vi "Initialize.vi"(8 "error in":errorcluster, 10 "InstanceName":string, 11 "Chiller Cluster - 2 Channel.lvclass":refnum<class "Climate Chamber - 2 Channel.lvclass">) -> (0 "error out":errorcluster, 3 "output cluster":refnum<class "Climate Chamber - 2 Channel.lvclass">)   [LabVIEW 2023, in "Climate Chamber - 2 Channel.lvclass"]
uses:
  Climate Chamber - 2 Channel.lvclass
  Climate Chamber - 2 Channel.lvclass/Climate Chamber - 2 Channel.ctl
  aa699e23-44e5-4879-a6c3-559a5ef9d2df.vi
  f052ae29-6a80-40ba-948a-362e912d77bd.vi
  293d8571-9b14-4487-9d38-5c4ef123197a.vi
  16278833-8dfa-4f0a-81f5-f65bd27da24d.vi
  da48c8f8-b897-4dcf-9451-5b341042a248.vi
  f0f9fcd1-ad99-4552-afb1-31be6853704b.vi
  aa699e23-44e5-4879-a6c3-559a5ef9d2df.vi/4bc1c15b-36ab-481f-b8dd-c64075ce723a.vi
  f052ae29-6a80-40ba-948a-362e912d77bd.vi/4bc1c15b-36ab-481f-b8dd-c64075ce723a.vi
  293d8571-9b14-4487-9d38-5c4ef123197a.vi/4bc1c15b-36ab-481f-b8dd-c64075ce723a.vi
  16278833-8dfa-4f0a-81f5-f65bd27da24d.vi/4bc1c15b-36ab-481f-b8dd-c64075ce723a.vi
  da48c8f8-b897-4dcf-9451-5b341042a248.vi/4bc1c15b-36ab-481f-b8dd-c64075ce723a.vi
  f0f9fcd1-ad99-4552-afb1-31be6853704b.vi/4bc1c15b-36ab-481f-b8dd-c64075ce723a.vi
  <vilib>/ADAS Replay HIL/Channels/Tag Wrapper/Polymorphic/Open Producer Tag (Cluster).vi
  <vilib>/ADAS Replay HIL/AdasHilServices/AdasHilServices Fill In Error Info Ex.vi
  <vilib>/ADAS Replay HIL/Channels/Tag Wrapper/Polymorphic/Open Consumer Tag (Cluster).vi
  Utilities/Utilities.lvlib
  <vilib>/ADAS Replay HIL/Channels/Tag Wrapper/Tag Wrapper.lvlib
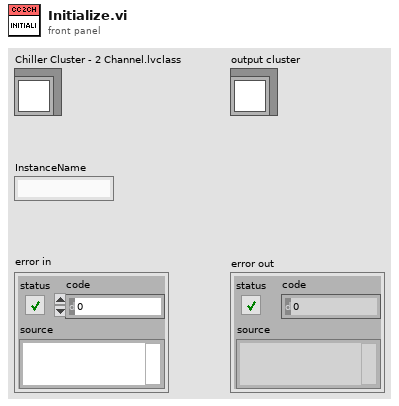
[diagram p1: front panel]
types:
  T1 = cluster{"OnOff.ACT":bool, "ErrorAcknowledge.ACT":bool}
  T2 = cluster{"OnOff.STS":i32, "Error.STS":i32, "Watchdog.STS":i32}
  T3 = cluster{"Temperature.ch01.SP":dbl, "TemperatureMIN.ch01.SP":dbl, "TemperatureMAX.ch01.SP":dbl, "TemperatureGrad.ch01.SP":dbl, "Humidity.ch01.SP":dbl, "HumidityMIN.ch01.SP":dbl, "HumidityMAX.ch01.SP":dbl, "HumidityGrad.ch01.SP":dbl}
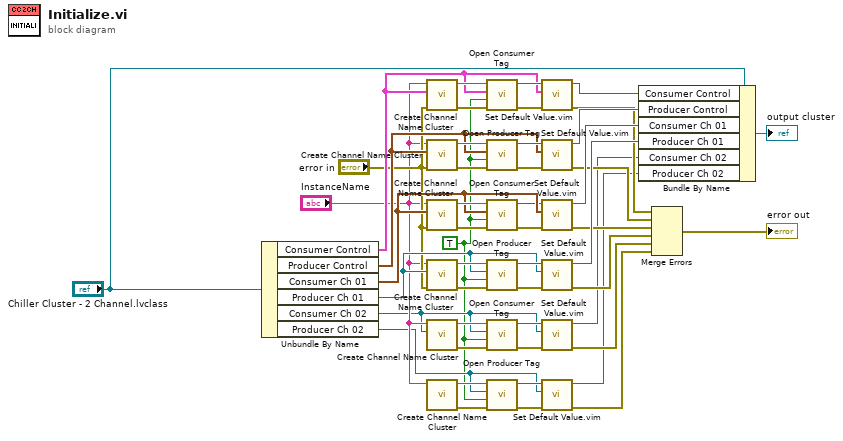
[diagram p0: block diagram]
diagram:
  w6 = TRUE ("Create if not found? (T)")
  n1 = Unbundle By Name("Chiller Cluster - 2 Channel.lvclass") -> ("Consumer Control"=w44:T1, "Producer Control"=w39:T2, "Consumer Ch 01"=w35:T3, "Producer Ch 01"=w31:refnum<k21>, "Consumer Ch 02"=w7:refnum<k21>, "Producer Ch 02"=w10:refnum<k21>)
  n2 = call "Create Channel Name Cluster.vi"("error in"="error in", "Cluster"=w44, "Instance Name"="InstanceName") -> ("error out"=w25:errorcluster, "Data Channel Name"=w48:string)  [unwired: 7 in]
  n3 = call "Create Channel Name Cluster.vi"("error in"="error in", "Cluster"=w39, "Instance Name"="InstanceName") -> ("error out"=w26:errorcluster, "Data Channel Name"=w47:string)  [unwired: 7 in]
  n4 = call "Create Channel Name Cluster.vi"("error in"="error in", "Cluster"=w35, "Instance Name"="InstanceName") -> ("error out"=w32:errorcluster, "Data Channel Name"=w38:string)  [unwired: 7 in]
  n5 = call "Create Channel Name Cluster.vi"("error in"="error in", "Cluster"=w31, "Instance Name"="InstanceName") -> ("error out"=w29:errorcluster, "Data Channel Name"=w37:string)  [unwired: 7 in]
  n6 = call "Create Channel Name Cluster.vi"("Cluster"=w7, "Instance Name"="InstanceName") -> ("error out"=w14:errorcluster, "Data Channel Name"=w9:string)  [unwired: 8 in]
  n7 = call "Create Channel Name Cluster.vi"("Instance Name"="InstanceName") -> ("error out"=w12:errorcluster, "Data Channel Name"=w17:string)  [unwired: 9 in]
  n8 = call-poly <vilib>:"Open Consumer Tag.vi"("error in"=w25, "Create if not found? (T)"=w6, "Cluster"=w44, "Channel Name"=w48) -> ("error out"=w43:errorcluster, "ADAS HIL Channel"=w46:refnum<k21>)  [unwired: 6 in]
  n9 = call-poly <vilib>:"Open Producer Tag.vi"("error in"=w26, "Create if not found? (T)"=w6, "Cluster"=w39, "Channel Name"=w47) -> ("error out"=w42:errorcluster, "ADAS HIL Channel"=w41:refnum<k21>)  [unwired: 6 in]
  n10 = call-poly <vilib>:"Open Consumer Tag.vi"("error in"=w32, "Create if not found? (T)"=w6, "Cluster"=w35, "Channel Name"=w38) -> ("error out"=w33:errorcluster, "ADAS HIL Channel"=w34:refnum<k21>)  [unwired: 6 in]
  n11 = call-poly <vilib>:"Open Producer Tag.vi"("error in"=w29, "Create if not found? (T)"=w6, "Cluster"=w31, "Channel Name"=w37) -> ("error out"=w30:errorcluster, "ADAS HIL Channel"=w36:refnum<k21>)  [unwired: 6 in]
  n12 = call-poly <vilib>:"Open Consumer Tag.vi"("error in"=w14, "Create if not found? (T)"=w6, "Cluster"=w7, "Channel Name"=w9) -> ("error out"=w15:errorcluster, "ADAS HIL Channel"=w8:refnum<k21>)  [unwired: 6 in]
  n13 = call-poly <vilib>:"Open Producer Tag.vi"("error in"=w12, "Create if not found? (T)"=w6, "Cluster"=w10, "Channel Name"=w17) -> ("error out"=w13:errorcluster, "ADAS HIL Channel"=w16:refnum<k21>)  [unwired: 6 in]
  n14 = call "Set Default Value.vim"("error in"=w43, "Data in"=w44, "ADAS HIL Channel in"=w46) -> ("error out"=w23:errorcluster, "ADAS HIL Channel out"=w45:refnum<k21>)  [unwired: 7 in]
  n15 = call "Set Default Value.vim"("error in"=w42, "Data in"=w39, "ADAS HIL Channel in"=w41) -> ("error out"=w22:errorcluster, "ADAS HIL Channel out"=w40:refnum<k21>)  [unwired: 7 in]
  n16 = call "Set Default Value.vim"("error in"=w33, "Data in"=w35, "ADAS HIL Channel in"=w34) -> ("error out"=w21:errorcluster, "ADAS HIL Channel out"=w28:refnum<k21>)  [unwired: 7 in]
  n17 = call "Set Default Value.vim"("error in"=w30, "Data in"=w31, "ADAS HIL Channel in"=w36) -> ("error out"=w20:errorcluster, "ADAS HIL Channel out"=w27:refnum<k21>)  [unwired: 7 in]
  n18 = call "Set Default Value.vim"("error in"=w15, "Data in"=w7, "ADAS HIL Channel in"=w8) -> ("error out"=w5:errorcluster, "ADAS HIL Channel out"=w3:refnum<k21>)  [unwired: 7 in]
  n19 = call "Set Default Value.vim"("error in"=w13, "Data in"=w10, "ADAS HIL Channel in"=w16) -> ("error out"=w4:errorcluster, "ADAS HIL Channel out"=w2:refnum<k21>)  [unwired: 7 in]
  n20 = Bundle By Name(cluster="Chiller Cluster - 2 Channel.lvclass", "Consumer Control"=w45, "Producer Control"=w40, "Consumer Ch 01"=w28, "Producer Ch 01"=w27, "Consumer Ch 02"=w3, "Producer Ch 02"=w2) -> (→"output cluster":refnum<class "Climate Chamber - 2 Channel.lvclass">)
  n21 = Merge Errors(w23, w22, w21, w20, w5, w4) -> (→"error out":errorcluster)
